vi "dfd_Check Integer MRate Filtering Mode.vi"(8 "error IO":errorcluster, 9 "filtering mode":T1 items=["No Rate Change", "Interpolation", "Decimation"]) -> (0 "error out":errorcluster)   [LabVIEW 2017, in "NI_DigFilterLicensed.lvlib"]
uses:
  <vilib>/addons/Digital Filter Design/NI_DigFilterLicensed.lvlib
  <vilib>/addons/Digital Filter Design/_Objects.llb/DFD Multirate Filtering Mode.ctl
  <vilib>/addons/Digital Filter Design/_Misc.llb/dfd_Error Handlers (Single).vi
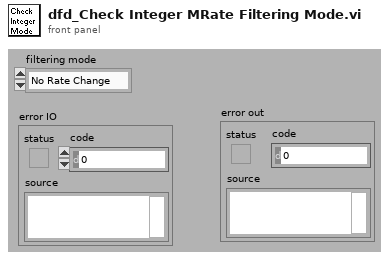
[diagram p1: front panel]
types:
  T1 = typedef "NI_DigFilterLicensed.lvlib/DFD Multirate Filtering Mode.ctl" = u16
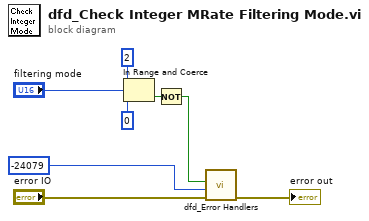
[diagram p0: block diagram]
diagram:
  n1 = In Range and Coerce(upper limit=u16 2, x="filtering mode", lower limit=u16 0) -> (In Range?=w7:bool)  [unwired: 1 out]
  n2 = Not(x=w7) -> (.not. x?=w8:bool)
  n3 = call-poly <vilib>:"dfd_Error Handlers.vi"("error in (no error)"="error IO", "error code"=-24079 ("ERR_FILTERING_MODE"), "condition failed?"=w8) -> ("error out"=→"error out":errorcluster)  [unwired: 8 out]
